vi "OutStation_Main.vi"(0 "Network Settings 1":T2={"port (20000)"=18000, "Master IP"="48.26.87.212", "Master Address"=12345, "Outstation Address "=54321, " update rate"=50}, 1 "Analog Input":dbl[](array[numeric]), 2 "Digital Input":bool[](array[boolean]), 5 "Settings Cluster":T1={"Default Variation:Analog Input Event (OBJ32)"=1, "Default Variation:Analog Input (OBJ30)"=1, "Default Variation:Binary Input (OBJ01)"=1, "Default Variation:Analog Output (OBJ40)"=4, "Default Variation:Binary Output Event (OBJ11)"=1, "Default Variation:Binary Output (OBJ10)"=1, "Default Variation:Analog Output Event (OBJ42)"=8, "Unsolicited Response Allowed"=FALSE, "Control:Select Timeout (ms)"=0, "Misc:Appl Confirmation Timeout"=0} {"Default Variation:Analog Output Event (OBJ42)" items=["32-bit without Time"=1, "16-bit without Time"=2, "32-bit with Time"=3, "16-bit with Time"=4, "Single-prec without Time"=5, "Double-prec without Time"=6, "Single-prec with Time"=7, "Double-prec with Time"=8]; "Default Variation:Binary Output (OBJ10)" items=["Packed Format"=1, "Output Status with Flags"=2]; "Default Variation:Binary Output Event (OBJ11)" items=["Status without Time"=1, "Status with Time"=2]; "Default Variation:Analog Output (OBJ40)" items=["32-bit with Flag"=1, "16-bit with Flag"=2, "Single-prec with Flag"=3, "Double-prec with Flag"=4]; "Default Variation:Binary Input (OBJ01)" items=["Packed Format"=1, "With Flags"=2]; "Default Variation:Analog Input (OBJ30)" items=["32-bit with Flag"=1, "16-bit with Flag"=2, "32-bit without Flag"=3, "16-bit without Flag"=4, "Single-prec with Flag"=5, "Double-prec with Flag"=6]; "Default Variation:Analog Input Event (OBJ32)" items=["32-bit without Time"=1, "16-bit without Time"=2, "32-bit with Time"=3, "16-bit with Time"=4, "Single-prec without Time"=5, "Double-prec without Time"=6, "Single-prec with Time"=7, "Double-prec with Time"=8]}, 7 "DNP3 DataMap 1":T3={"Binary Output Points"=1, "Binary Input Points"=0, "Analog Output Points"=20, "Analog Input Points"=20}, 9 "OS_Reset":bool, 11 "OS_Enable":bool, 12 "DNP3 Session Input":T4) -> (3 "Analog Output":dbl[](array[numeric]), 4 "OS_DNP3_Settings_Changed":bool, 6 "Analog Changed":bool[](array[boolean]), 8 "Connected?":bool, 10 "Digital Changed":bool[](array[boolean]), 14 "DNP3 Session":T4, 15 "Digital Output":T5[](array[typedef]) {"Control" items=["Nul"=0, "Pulse On"=1, "Pulse Off"=2, "Latch On"=3, "Latch Off"=4, "Close"=65, "Trip"=129]})   [LabVIEW 2016]
uses:
  <vilib>/DNP3/DNP3_Common/crob.ctl
  <vilib>/DNP3/DNP3_Common/crob_ctrl.ctl
  <vilib>/DNP3/DNP3_Outstation/Write Binary Input.vi
  <vilib>/DNP3/DNP3_Outstation/Read Binary Output.vi
  <vilib>/DNP3/DNP3_Outstation/Write Analog Input.vi
  <vilib>/DNP3/DNP3_Outstation/Read Analog Output.vi
  <vilib>/DNP3/DNP3_Common/Create Channel (IP Networking).vi
  <vilib>/DNP3/DNP3_Common.lvlib
  <vilib>/DNP3/DNP3_Outstation.lvlib
  <resource>/objmgr/dnp3.rc
panel:
  out "Array 2":u8[](array[numeric])
  out "OS_Reset_Succesful":bool
  out "OS_Reset_Ind":bool
  out "OS_DNP3_Settings_Initial":T1
  out "OS_Network_Settings_Initial":T2
  out "DNP3 DataMap_Initial":T3={"Binary Output Points"=1, "Binary Input Points"=0, "Analog Output Points"=7, "Analog Input Points"=6}
  out "x > y?":bool
  out "Analog Input Points":u16 max=32
  out "Analog Output Points":u16 max=32
  out "Binary Input Points":u16 max=32
  out "Binary Output Points":u16 max=32
  out "Reset Cycles":i32
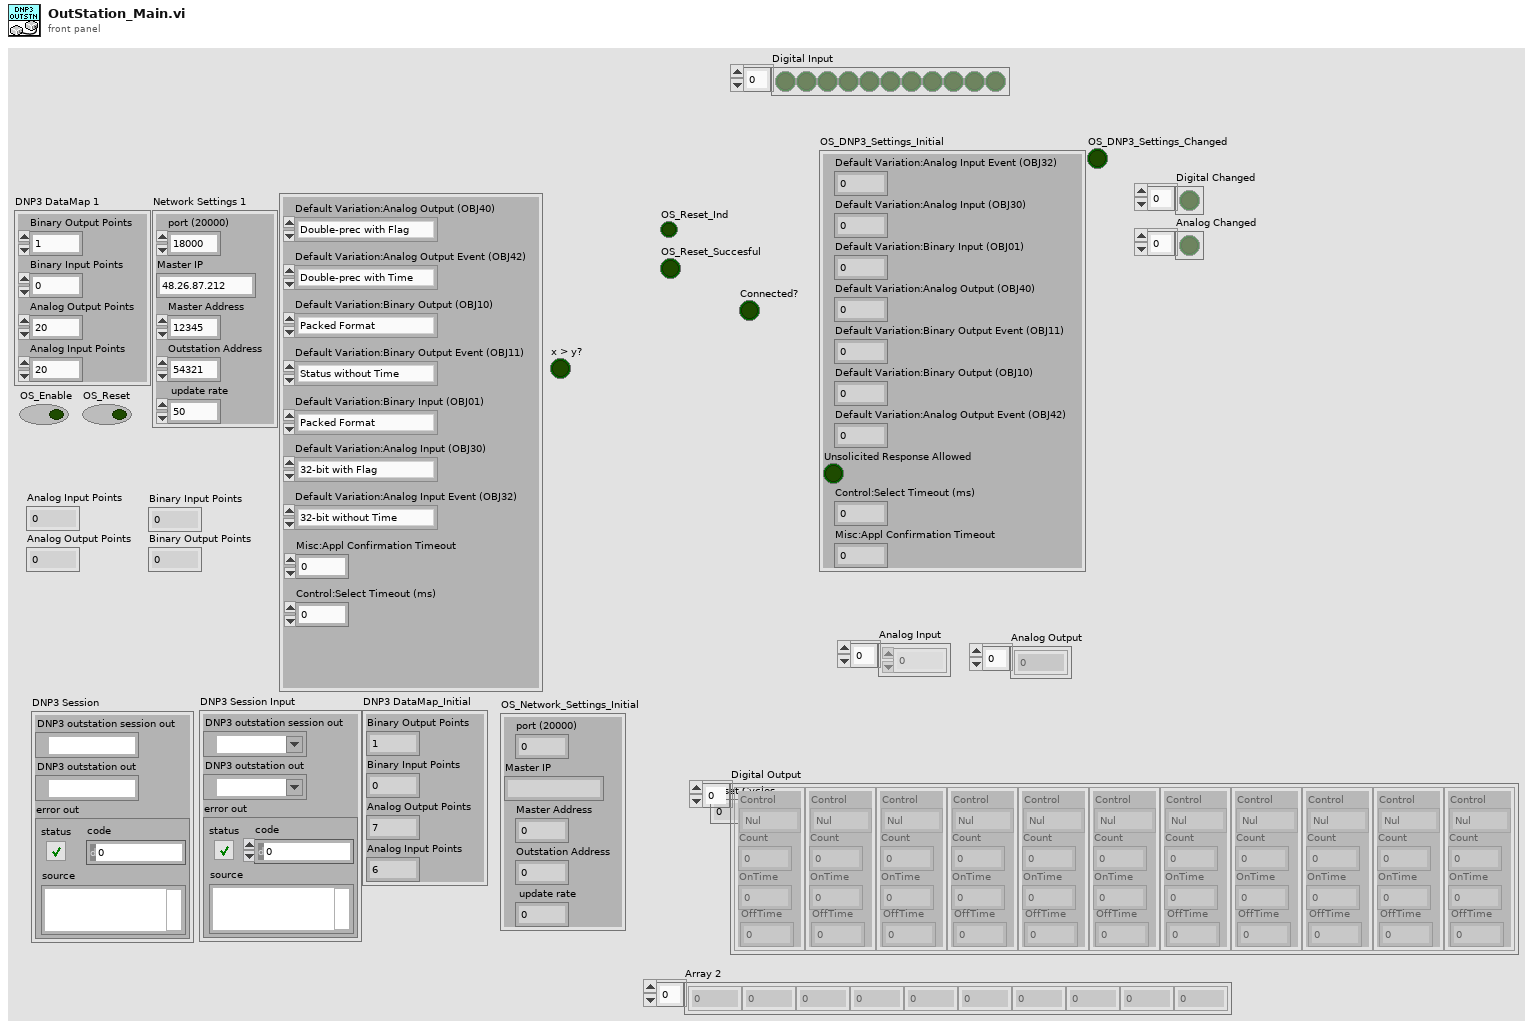
[diagram p1: front panel]
types:
  T1 = cluster{"Default Variation:Analog Input Event (OBJ32)":u8, "Default Variation:Analog Input (OBJ30)":u8, "Default Variation:Binary Input (OBJ01)":u8, "Default Variation:Analog Output (OBJ40)":u8, "Default Variation:Binary Output Event (OBJ11)":u8, "Default Variation:Binary Output (OBJ10)":u8, "Default Variation:Analog Output Event (OBJ42)":u8, "Unsolicited Response Allowed":bool, "Control:Select Timeout (ms)":u32, "Misc:Appl Confirmation Timeout":u32}
  T2 = cluster{"port (20000)":u16, "Master IP":string, "Master Address":u16, "Outstation Address ":u16, " update rate":u32}
  T3 = cluster{"Binary Output Points":u16, "Binary Input Points":u16, "Analog Output Points":u16, "Analog Input Points":u16}
  T4 = cluster{"DNP3 outstation session out":refnum<k21>, "DNP3 outstation out":refnum<k21>, "error out":errorcluster}
  T5 = typedef "DNP3_Common.lvlib/crob.ctl" = cluster{"OnTime":u32, "Count":u8, "OffTime":u32, "Control":T6}
  T6 = typedef "DNP3_Common.lvlib/crob_ctrl.ctl" = u8
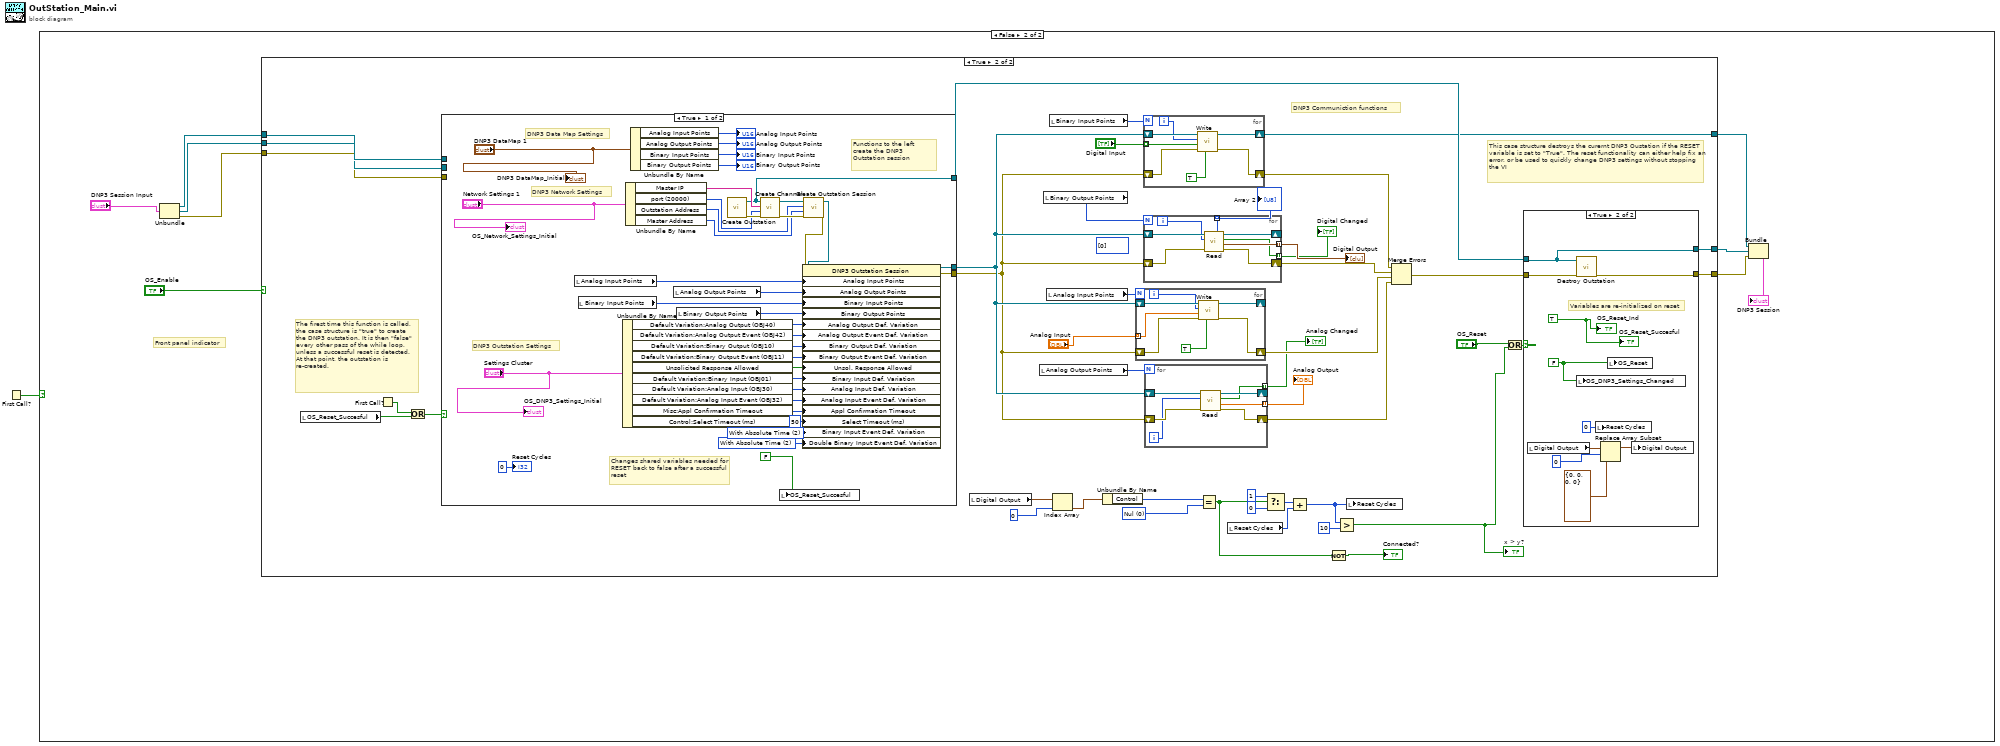
[diagram p0: block diagram]
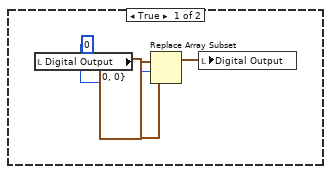
[diagram p2: hidden frame]
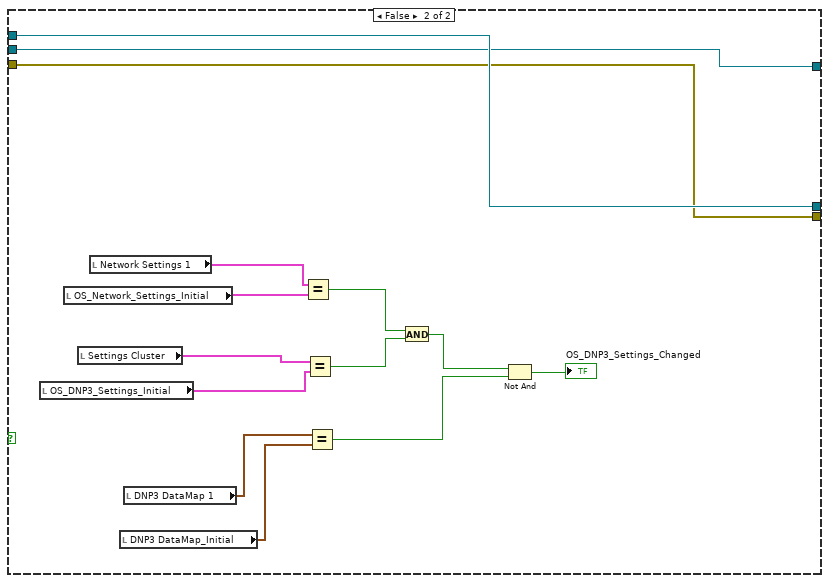
[diagram p5: hidden frame]
diagram:
  n1 = First Call?() -> (First Call?: T/F=w1:bool)
  n2 = case shown="False" w1 {
    frame True {
      n3 = local read "Digital Output"() -> (w3:T5[])
      n4 = Replace Array Subset(array=w3, new element=T5 {"OnTime"=0, "Count"=0, "OffTime"=0, "Control"=0} ("new element/subarray"), index=0) -> (w2:T5[])
      n5 = local write "Digital Output"(w2) -> ()
    }
    frame False {
      # "Front panel indicator"
      n6 = Unbundle("DNP3 Session Input") -> ("DNP3 outstation session out"=w8:refnum<k21>, "DNP3 outstation out"=w7:refnum<k21>, "error out"=w6:errorcluster)
      n7 = case shown="True" "OS_Enable" {
        tunnel: w8 -> [w17 w55]
        tunnel: w7 -> [w16 w54]
        tunnel: [w17 w21] -> w13
        tunnel: [w16 w53] -> w12
        tunnel: [w15 w52] -> w11
        tunnel: w6 -> [w15 w51]
        frame False {
        }
        frame True {
          (unwired) u16[] [0] ("Array")
          w46 = T6 0 items=["Nul"=0, "Pulse On"=1, "Pulse Off"=2, "Latch On"=3, "Latch Off"=4, "Close"=65, "Trip"=129] ("y")
          # "DNP3 Communiction functions"
          # "This case structure destroys the curernt DNP3 Oustation if the RESET variable is set to \"True\". The reset functionality can either help fix an error, or be used to quickly change DNP3 settings without stopping the VI"
          # "The firest time this function is called, the case structure is \"true\" to create the DNP3 outstation. It is then \"false\" every other pass of the while loop, unless a successful reset is detected. At that point, the outstation is re-created."
          n8 = local read "OS_Reset_Succesful"() -> (w26:bool)
          n9 = First Call?() -> (First Call?: T/F=w56:bool)
          n10 = Or(x=w56, y=w26) -> (x .or. y?=w57:bool)
          n11 = case shown="True" w57 {
            tunnel: [w116 w153] -> w61
            tunnel: [w115 w151] -> w60
            tunnel: [w114 w152] -> w59
            tunnel: w55 -> [_ w153]
            tunnel: w54 -> [_ w152]
            tunnel: w51 -> [_ w151]
            frame True {
              w105 = u8 2 items=["Without Time"=1, "With Absolute Time"=2, "With Relative Time"=3] ("Default Variation:Double Binary Input Event (OBJ04)")
              w106 = u8 2 items=["Without Time"=1, "With Absolute Time"=2, "With Relative Time"=3] ("Default Variation:Binary Input Event (OBJ02)")
              # "Functions to the left create the DNP3 Outstation session"
              # "DNP3 Data Map Settings"
              # "DNP3 Network Settings"
              # "DNP3 Outstation Settings"
              # "Changes shared variables needed for RESET back to false after a successful reset"
              n12 = local read "Analog Input Points"() -> (w117:u16)
              n13 = local read "Binary Input Points"() -> (w119:u16)
              n14 = Unbundle By Name("Settings Cluster") -> ("Default Variation:Analog Output (OBJ40)"=w121:u8, "Default Variation:Analog Output Event (OBJ42)"=w122:u8, "Default Variation:Binary Output (OBJ10)"=w123:u8, "Default Variation:Binary Output Event (OBJ11)"=w124:u8, "Unsolicited Response Allowed"=w104:bool, "Default Variation:Binary Input (OBJ01)"=w125:u8, "Default Variation:Analog Input (OBJ30)"=w126:u8, "Default Variation:Analog Input Event (OBJ32)"=w127:u8, "Misc:Appl Confirmation Timeout"=w128:u32)  [unwired: 1 out]
              n15 = Unbundle By Name("Network Settings 1") -> ("Master IP"=w136:string, "port (20000)"=w135:u16, "Outstation Address"=w134:u16, "Master Address"=w133:u16)
              n16 = Unbundle By Name("DNP3 DataMap 1") -> ("Analog Input Points"=→"Analog Input Points":u16, "Analog Output Points"=→"Analog Output Points":u16, "Binary Input Points"=→"Binary Input Points":u16, "Binary Output Points"=→"Binary Output Points":u16)
              n17 = local read "Analog Output Points"() -> (w118:u16)
              n18 = local read "Binary Output Points"() -> (w120:u16)
              n19 = call <vilib>:"Create Outstation.vi"() -> ("error out"=w139:errorcluster, "DNP3 outstation out"=w114:refnum<k21>)  [unwired: 10 in]
              n20 = call-poly <vilib>:"Create Channel.vi"("error in (no error)"=w139, "port (20000)"=w135, "IP"=w136, "DNP3 outstation"=w114) -> ("error out"=w138:errorcluster, "DNP3 channel out"=w137:refnum<k21>)  [unwired: 6 in]
              n21 = local write "OS_Reset_Succesful"(FALSE ("Reset Outstation")) -> ()
              n22 = call <vilib>:"Create Outstation Session.vi"("error in (no error)"=w138, "destination"=w133, "source"=w134, "DNP3 channel"=w137) -> ("error out"=w108:errorcluster, "DNP3 outstation session out"=w107:refnum<k21>)  [unwired: 6 in]
              n23 = property class="DNP3 Outstation Session"(reference=w107, error in=w108, "Analog Input Points"=w117, "Analog Output Points"=w118, "Binary Input Points"=w119, "Binary Output Points"=w120, "Analog Output Def. Variation"=w121, "Analog Output Event Def. Variation"=w122, "Binary Output Def. Variation"=w123, "Binary Output Event Def. Variation"=w124, "Unsol. Response Allowed"=w104, "Binary Input Def. Variation"=w125, "Analog Input Def. Variation"=w126, "Analog Input Event Def. Variation"=w127, "Appl Confirmation Timeout"=w128, "Select Timeout (ms)"=u32 50 ("Control:Select Timeout (ms)"), "Binary Input Event Def. Variation"=w106, "Double Binary Input Event Def. Variation"=w105) -> (reference out=w116:refnum<k21>, error out=w115:errorcluster)
              "Reset Cycles" <- 0 ("Reset Cycles")
              "DNP3 DataMap_Initial" <- "DNP3 DataMap 1"
              "OS_Network_Settings_Initial" <- "Network Settings 1"
              "OS_DNP3_Settings_Initial" <- "Settings Cluster"
            }
            frame False {
              n24 = local read "OS_DNP3_Settings_Initial"() -> (w142:T1)
              n25 = local read "OS_Network_Settings_Initial"() -> (w141:T2)
              n26 = local read "Settings Cluster"() -> (w143:T1)
              n27 = local read "Network Settings 1"() -> (w140:T2)
              n28 = local read "DNP3 DataMap_Initial"() -> (w144:T3)
              n29 = local read "DNP3 DataMap 1"() -> (w145:T3)
              n30 = Equal?(x=w140, y=w141) -> (x = y?=w149:bool)
              n31 = Equal?(x=w143, y=w142) -> (x = y?=w148:bool)
              n32 = Equal?(x=w145, y=w144) -> (x = y?=w150:bool)
              n33 = And(x=w149, y=w148) -> (x .and. y?=w147:bool)
              n34 = Not And(1:w150, 2:w147) -> (0:→"OS_DNP3_Settings_Changed":bool)
            }
          }
          n35 = local read "Digital Output"() -> (w41:T5[])
          n36 = local read "Analog Output Points"() -> (w32:u16)
          n37 = local read "Binary Output Points"() -> (w34:u16)
          n38 = local read "Analog Input Points"() -> (w33:u16)
          n39 = local read "Binary Input Points"() -> (w35:u16)
          n40 = Index Array(array=w41, index=0) -> (element=w39:T5)
          n41 = Unbundle By Name(w39) -> ("Control"=w38:T6)
          n42 = for {
            N: w33 -> [_]
            shift-right: [w80] -> w29
            shift-left: w60 -> [w81]
            shift-right: [w82] -> _
            shift-left: w61 -> [w83]
            tunnel: "Analog Input" -> [w78] mode=indexing
            i -> [w77]
            n43 = call-poly <vilib>:"Write.vi"("generate event? (false)"=TRUE, "error in (no error)"=w81, "value"=w78, "point index"=w77, "DNP3 outstation session"=w83) -> ("error out"=w80:errorcluster, "DNP3 outstation session"=w82:refnum<k21>)  [unwired: 5 in]
          }
          n44 = for {
            N: w35 -> [_]
            shift-right: [w89] -> w21
            shift-left: w61 -> [w90]
            shift-right: [w87] -> w31
            shift-left: w60 -> [w88]
            tunnel: "Digital Input" -> [w85] mode=indexing
            i -> [w86]
            n45 = call-poly <vilib>:"Write.vi"("generate event? (false)"=TRUE, "error in (no error)"=w88, "value"=w85, "point index"=w86, "DNP3 outstation session"=w90) -> ("error out"=w87:errorcluster, "DNP3 outstation session"=w89:refnum<k21>)  [unwired: 5 in]
          }
          n46 = for {
            N: w34 -> [_]
            shift-right: [w76] -> _
            shift-left: w61 -> [w75]
            shift-right: [w73] -> w30
            shift-left: w60 -> [w74]
            tunnel: [w72] -> w23 mode=indexing
            tunnel: [w70] -> w19 mode=indexing
            tunnel: [w69] -> w20 mode=indexing
            i -> [w71]
            n47 = call-poly <vilib>:"Read.vi"("error in (no error)"=w74, "point index"=w71, "DNP3 outstation session"=w75) -> ("error out"=w73:errorcluster, "CROB value"=w72:T5, "changed?"=w70:bool, "DNP3 outstation session"=w76:refnum<k21>, "object flags"=w69:u8)  [unwired: 4 in]
          }
          "Digital Output" <- w23
          "Array 2" <- w20
          "Digital Changed" <- w19
          n48 = for {
            N: w32 -> [_]
            shift-right: [w66] -> _
            shift-left: w61 -> [w67]
            shift-right: [w64] -> w28
            shift-left: w60 -> [w65]
            tunnel: [w68] -> w27 mode=indexing
            tunnel: [w62] -> w18 mode=indexing
            i -> [w63]
            n49 = call-poly <vilib>:"Read.vi"("error in (no error)"=w65, "point index"=w63, "DNP3 outstation session"=w67) -> ("error out"=w64:errorcluster, "current value"=w68:dbl, "changed?"=w62:bool, "DNP3 outstation session"=w66:refnum<k21>)  [unwired: 4 in, 1 out]
          }
          "Analog Output" <- w27
          "Analog Changed" <- w18
          n50 = Equal?(x=w38, y=w46) -> (x = y?=w42:bool)
          n51 = local read "Reset Cycles"() -> (w45:i32)
          n52 = Select(t=1, s=w42, f=0) -> (s? t:f=w47:i32)
          n53 = Add(x=w47, y=w45) -> (x+y=w43:i32)
          n54 = Not(x=w42) -> (.not. x?=→"Connected?":bool)
          n55 = Greater?(x=w43, y=10) -> (0:w37:bool)
          "x > y?" <- w37
          n56 = local write "Reset Cycles"(w43) -> ()
          n57 = Merge Errors(w31, w30, w29, w28) -> (w58:errorcluster)
          n58 = Or(x="OS_Reset", y=w37) -> (x .or. y?=w50:bool)
          n59 = case shown="True" w50 {
            tunnel: w59 -> [w91 w100]
            tunnel: w58 -> [w92 w102]
            tunnel: [w92 w101] -> w52
            tunnel: [w91 w100] -> w53
            frame False {
            }
            frame True {
              w93 = FALSE ("Comm_Reset")
              w94 = TRUE ("OS1 TX/RX 2")
              # "Variables are re-initialized on reset"
              n60 = local read "Digital Output"() -> (w97:T5[])
              n61 = local write "OS_DNP3_Settings_Changed"(w93) -> ()
              n62 = call <vilib>:"Destroy Outstation.vi"("error in (no error)"=w102, "DNP3 outstation"=w100) -> ("error out"=w101:errorcluster)  [unwired: 9 in]
              n63 = local write "Reset Cycles"(0 ("Reset Cycles")) -> ()
              n64 = Replace Array Subset(array=w97, new element=T5 {"OnTime"=0, "Count"=0, "OffTime"=0, "Control"=0} ("new element/subarray"), index=0) -> (w98:T5[])
              n65 = local write "OS_Reset"(w93) -> ()
              n66 = local write "Digital Output"(w98) -> ()
              "OS_Reset_Ind" <- w94
              "OS_Reset_Succesful" <- w94
            }
          }
        }
      }
      n67 = Bundle("DNP3 outstation session out"=w13, "DNP3 outstation out"=w12, "error out"=w11) -> (→"DNP3 Session":T4)  [unwired: 1 in]
    }
  }
